vi "StringToHex.vi"(11 "STRING":string) -> (3 "数组":u16[](array[numeric]) format="%04xH")   [LabVIEW 2016, in "斯坦道CODMn.lvlib"]
panel:
  out "无符号字节数组":u8[](array[numeric]) format="%xH"
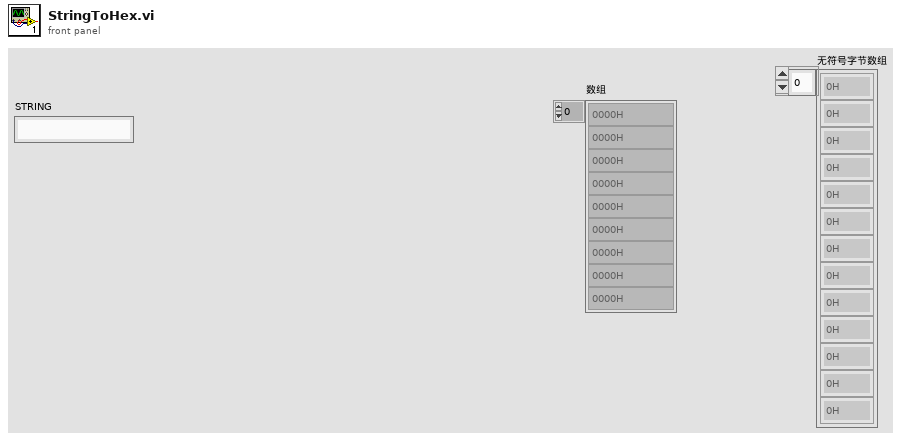
[diagram p1: front panel]
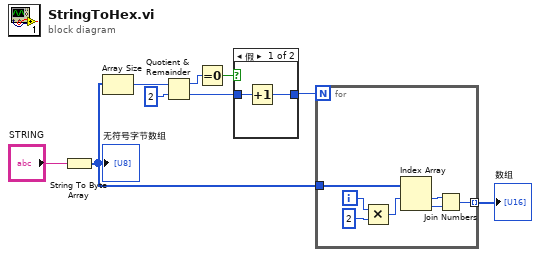
[diagram p0: block diagram]
diagram:
  n1 = String To Byte Array(string="STRING") -> (unsigned byte array=w1:u8[])
  "无符号字节数组" <- w1
  n2 = Array Size(array=w1) -> (size(s)=w8:i32)
  n3 = Quotient & Remainder(x=w8, y=2) -> (x-y*floor(x/y)=w6:i32, floor(x/y)=w4:i32)
  n4 = Equal To 0?(x=w6) -> (x = 0?=w5:bool)
  n5 = case shown="假" w5 {
    tunnel: [w10 w12] -> w3
    tunnel: w4 -> [w11 w12]
    frame False {
      n6 = Increment(x=w11) -> (x+1=w10:i32)
    }
    frame True {
    }
  }
  n7 = for {
    N: w3 -> [_]
    tunnel: w1 -> [w19]
    tunnel: [w13] -> w2 mode=indexing
    i -> [w18]
    n8 = Multiply(x=w18, y=2) -> (x*y=w16:i32)
    n9 = Index Array(array=w19, index #1=w16) -> (element #1=w15:u8, element #2=w14:u8)  [unwired: 1 in]
    n10 = Join Numbers(hi=w15, lo=w14) -> ((hi.lo)=w13:u16)
  }
  "数组" <- w2
